vi "realtime-callable-func.vi"() -> ()   [LabVIEW 2018]
uses:
  <vilib>/Platform/TimedLoop/XDataNode/timing_clust.ctl
  <vilib>/Platform/TimedLoop/XDataNode/nitl_modes.ctl
  <vilib>/Platform/TimedLoop/XDataNode/wakeup.ctl
  <vilib>/rvi/Emulation/niFpgaGetClockAttributes.vi
  <vilib>/rvi/Emulation/niFpgaSctlEmulationGetInTimedLoop.vi
  <vilib>/rvi/Emulation/niFpgaEmulationReportErrorSimple.vi
  <vilib>/rvi/Emulation/niFpgaProcessEmulError.vi
  <vilib>/rvi/Emulation/niFpgaCriticalErrorInLSC.vi
  <vilib>/Platform/TimedLoop/XDataNode/XDataNode.xnode
  <vilib>/Platform/TimedLoop/XDataNode/XDNodeRunTimeDep.lvlib
panel:
  out "x != y?":bool
  out "32bit integer":i32
  out "s? t:f":fxp<+/-,32,16>
  in  "stop":bool
  out "ready for input":bool
  in  "Input":fxp<+/-,32,16>
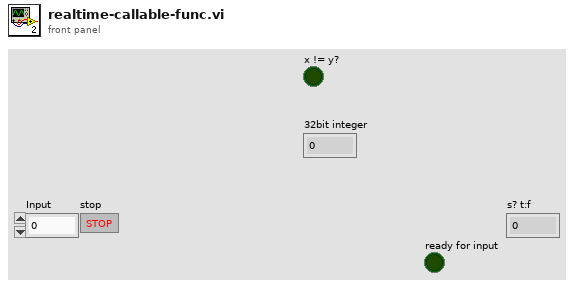
[diagram p1: front panel]
types:
  T1 = typedef "XDNodeRunTimeDep.lvlib/timing_clust.ctl" = cluster{"Expected End [f-1]":u64, "Actual End [f-1]":u64, "Finished Late? [f-1]":bool, "Expected End [i-1]":u64, "Actual End [i-1]":u64, "Finished Late? [i-1]":bool, "Expected Start [i]":u64, "Actual Start [i]":u64, "Expected Start [f]":u64, "Actual Start [f]":u64, "Source Name":string, "Structure Name":string, "Period":i64, "Deadline":i64, "Offset":i64, "Start":i64, "Priority":i32, "Timeout":i32, "Mode":T2, "Wakeup Reason":T3, "Error":errorcluster, "Source Type":string, "Secondary Source Type":string, "Global End Time":u64, "Global Start Time":u64, "Frame Duration":u64, "Iteration Duration":u64, "Assigned CPU":i32, "I/O Scan Engine Mode":u32}
  T2 = typedef "XDNodeRunTimeDep.lvlib/nitl_modes.ctl" = enum32{"No Change", "Process missed periods, maintain original phase", "Discard missed periods, maintain original phase", "Process missed periods, ignore original phase", "Discard missed periods, ignore original phase"}
  T3 = typedef "XDNodeRunTimeDep.lvlib/wakeup.ctl" = enum32{"Normal", "Aborted", "Asynchronous wakeup", "Timing source error", "Timed loop error", "Timeout"}
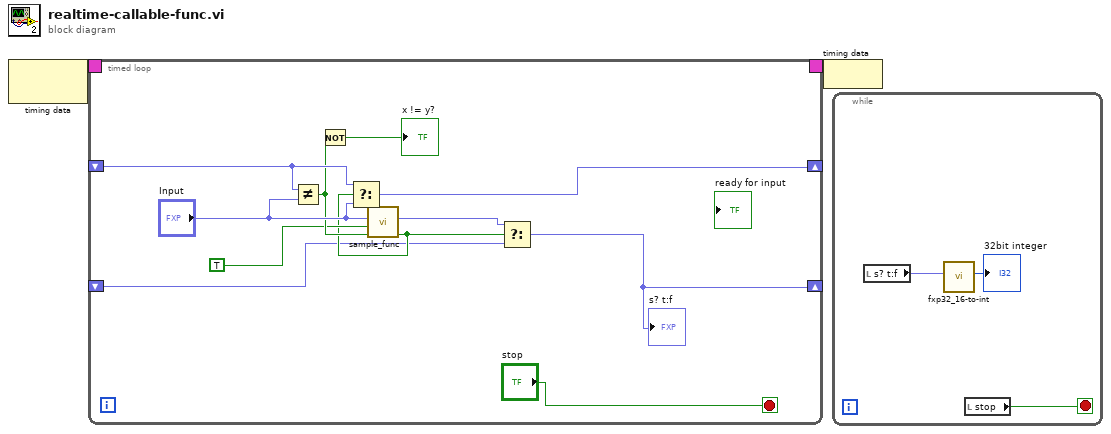
[diagram p0: block diagram]
diagram:
  n1 = node-c288() -> (w2:T1)  [unwired: 1 in]
  n2 = timed-loop {
    timing: w2 -> [_]
    timing-out: [_] -> w1
    shift-right: [w4] -> _
    shift-left: _ -> [w5]
    shift-right: [w7] -> _
    shift-left: _ -> [w12]
    stop <- "stop" stop-if-true
    n3 = Not Equal?(x=w12, y="Input") -> (x != y?=w10:bool)
    n4 = Not(x=w10) -> (.not. x?=→"x != y?":bool)
    n5 = call "sample_func.vi"("input valid"=w10, "ready for output (T)"=TRUE, "x"="Input") -> ("output valid"=w8:bool, "Output"=w6:fxp<+/-,32,16>)  [unwired: 6 in, 1 out]
    n6 = Select(t=w12, s=w8, f="Input") -> (s? t:f=w7:fxp<+/-,32,16>)
    n7 = Select(t=w6, s=w8, f=w5) -> (s? t:f=w4:fxp<+/-,32,16>)
    "s? t:f" <- w4
  }
  n8 = node-c288(w1) -> ()
  n9 = while {
    stop <- w18 stop-if-true
    n10 = local read "s? t:f"() -> (w17:fxp<+/-,32,16>)
    n11 = call "fxp32_16-to-int.vi"("FXP32_16"=w17) -> ("32bit integer"=→"32bit integer":i32)  [unwired: 10 in]
    n12 = local read "stop"() -> (w18:bool)
  }
